vi "mtlb simx Auxiliary Console Open.vi"(0 "clientIDandMaxLinesAndModeAndPositionAndSize":i32, 1 "consoleHandle":i32, 5 "title":string, 7 "textColor":sgl, 9 "backgroundColor":sgl, 11 "error in (no error)":errorcluster, 12 "operationMode":i32) -> (3 "consoleHandle out":i32, 4 "clientIDandMaxLinesAndModeAndPositionAndSize out":i32, 6 "function return":i32, 8 "textColor out":sgl, 10 "backgroundColor out":sgl, 15 "error out":errorcluster)   [LabVIEW 2019, in "PXL_V-REP.lvlib"]
doc: "EXTAPI_DLLEXPORT simxInt mtlb_simxAuxiliaryConsoleOpen(simxInt* clientIDandMaxLinesAndModeAndPositionAndSize,const simxChar* title,simxFloat* textColor,simxFloat* backgroundColor,simxInt* consoleHandle,simxInt operationMode);"
uses:
  PXL_V-REP.lvlib
  <userlib>/V-REP/remoteApi.dll
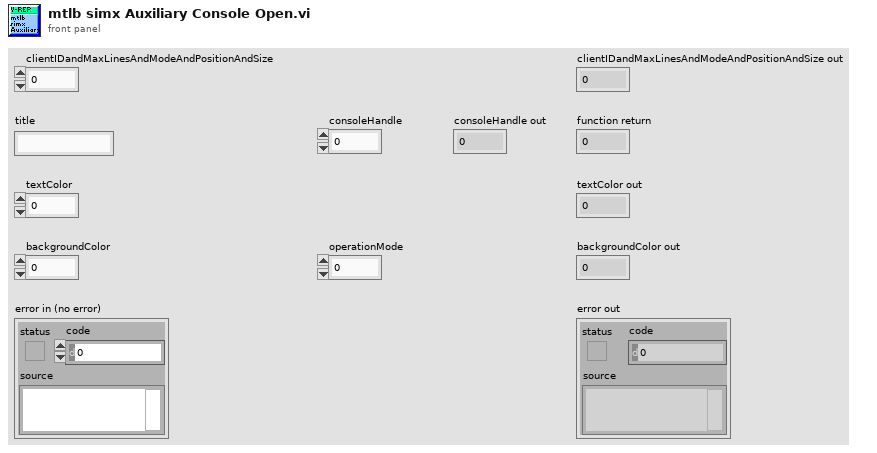
[diagram p1: front panel]
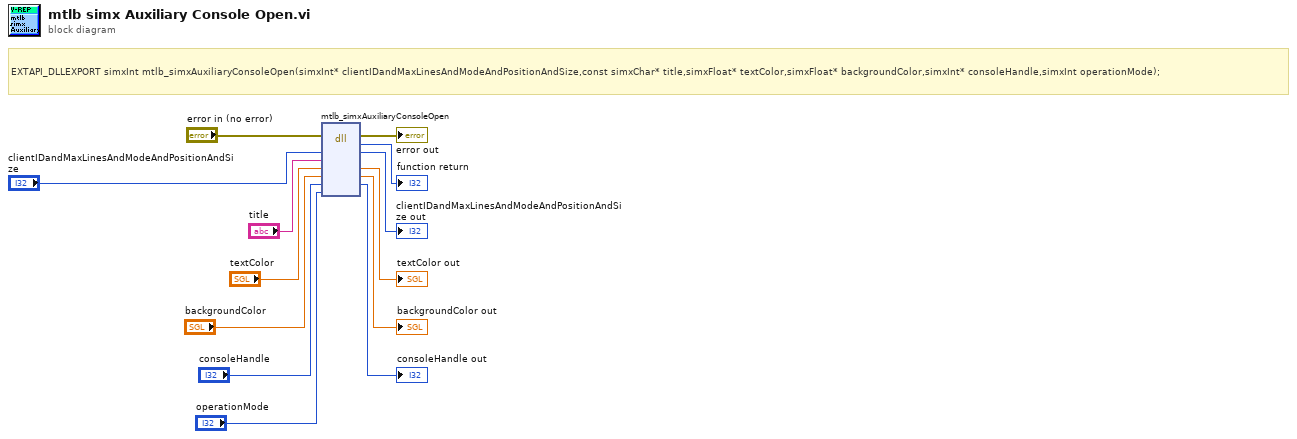
[diagram p0: block diagram]
diagram:
  # "EXTAPI_DLLEXPORT simxInt mtlb_simxAuxiliaryConsoleOpen(simxInt* clientIDandMaxLinesAndModeAndPositionAndSize,const simxChar* title,simxFloat* textColor,simxFloat* backgroundColor,simxInt* consoleHandle,simxInt operationMode);"
  n1 = dll-call lib="C:/Program Files (x86)/National Instruments/LabVIEW 2019/user.lib/V-REP/remoteApi.*" fn="mtlb_simxAuxiliaryConsoleOpen"(error in="error in (no error)", "clientIDandMaxLinesAndModeAndPositionAndSize"="clientIDandMaxLinesAndModeAndPositionAndSize", "title"="title", "textColor"="textColor", "backgroundColor"="backgroundColor", "consoleHandle"="consoleHandle", "operationMode"="operationMode") -> (error out=→"error out":errorcluster, →"function return":i32, "clientIDandMaxLinesAndModeAndPositionAndSize"=→"clientIDandMaxLinesAndModeAndPositionAndSize out":i32, "textColor"=→"textColor out":sgl, "backgroundColor"=→"backgroundColor out":sgl, "consoleHandle"=→"consoleHandle out":i32)  [unwired: 4 in, 1 out]
